vi "intialize_bottom_cam (SubVI).vi"(0 "Gain":sgl, 5 "Exposure time (ms)":sgl) -> (3 "images array out":u8[](array[numeric]), 6 "Handle out":u64, 10 "BGR out":u8[](array[numeric]), 14 "Pixel Format":u32, 15 "error out":errorcluster)   [LabVIEW 2016]
uses:
  <userlib>/Lumenera/NiLuApi.lvlibp/Controls/LuProp.ctl
  <userlib>/Lumenera/NiLuApi.lvlibp
panel:
  out "frameRate out":sgl
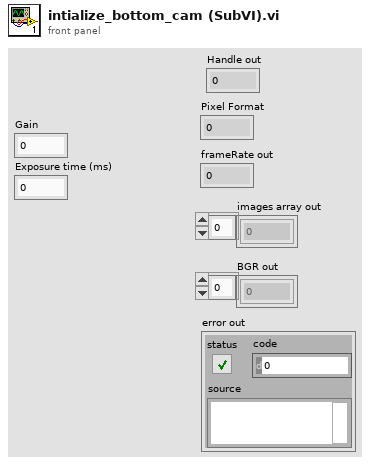
[diagram p1: front panel]
types:
  T1 = typedef "NiLuApi.lvlibp/LuProp.ctl" = u32
  T2 = cluster{"X Offset":u32, "Y Offset":u32, "Width":u32, "Heigth":u32, "Pixel Format":u32, "Bin/Sub X":u16, "FLags X":u16, "Bin/Sub Y":u16, "Flags Y":u16}
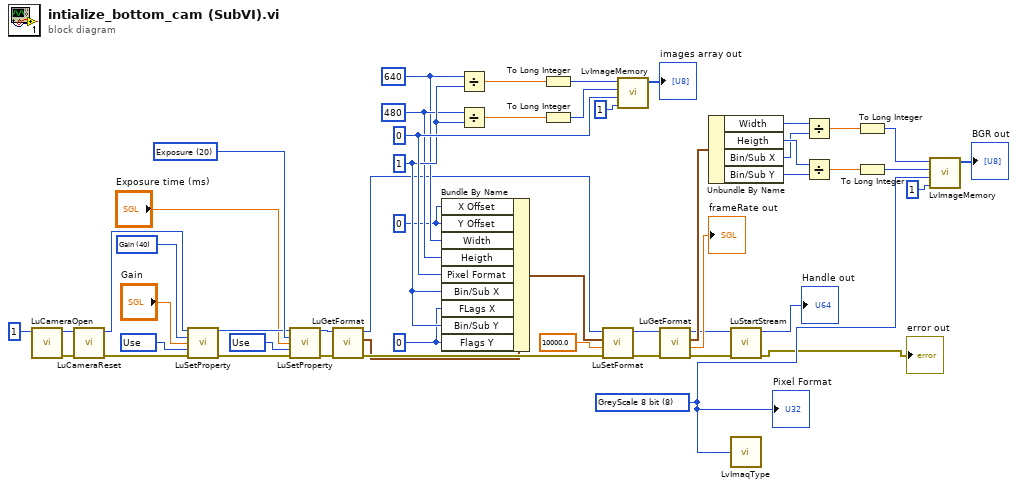
[diagram p0: block diagram]
diagram:
  w32 = u32 8 items=["8 Bit raw", "16 Bit raw", "RGB 24", "YUV422", "COUNT", "FILTER", "RGB 32", "RGB 48", "GreyScale 8 bit", "GreyScale 16 bit"] ("Pixel Format")
  w27 = u32 0 ("Pixel Format")
  w20 = u32 640 ("Width")
  w21 = u32 480 ("Heigth")
  w14 = u32 0 ("X Offset")
  w22 = u16 1 ("Bin/Sub X")
  w13 = u16 0 ("FLags X")
  w9 = -2147483648 items=["None"=0, "Use"=-2147483648, "Auto\\Master\\Little Endian"=1073741824, "Strobe From Start of Exposure"=536870912, "Polarity"=268435456, "Memory Readback"=134217728, "Unknown Maximum"=131072, "Unknown Minimum"=65536, "Red"=1, "Green1"=2, "Green2"=4, "Blue"=8] ("Capability Flag")
  w7 = T1 20 items=["Contrast"=1, "Hue"=2, "Brightness"=0, "Saturation"=3, "Sharpness"=4, "Gamma"=5, "Pan"=16, "Tilt"=17, "Roll"=18, "Zoom"=19, "Exposure"=20, "Iris"=21, "Focus"=22, "Gain"=40, "Gain Red/Magenta"=41, "Gain Blue/Cyan"=42, "Gain Green1/Yellow1"=43, "Gain Green2/Yellow2"=44, "Still Exposure"=50, "Still Gain"=51, "Red Still Gain"=52, "Green1 Still Gain"=53, "Green2 Still Gain"=54, "Blue Still Gain"=55, "Still Strobe Delay"=56, "Still Exposure Delay"=100, "Demosaicing Method"=64, "Correction Matrix"=65, "Flipping"=66, "Digital Whitebalance U"=69, "Digital Whitebalance V"=70, "Digital Gain"=71, "Digital Gain Red"=72, "Digital Gain Green"=73, "Digital Gain Blue"=74, "Color Format"=80, "Max Width"=81, "Max Height"=82, "ABS Focus"=85, "Black Level"=86, "Still Knee1 Exposure"=96, "Still Knee2 Exposure"=97, "Still Knee3 Exposure"=98, "Video Knee"=99, "Threshold"=101, "Auto Exp Target"=103, "Timestamps"=105, "Snapshot Clock Speed"=106, "Auto Exp Maximum"=107, "Temperature"=108, "Trigger"=110, "Frame Gate"=112, "Exposure Interval"=113, "PWM"=114, "Memory"=115, "Still Strobe Duration"=116, "Fan"=118, "Sync Mode"=119, "Snapshot Count"=120, "LSC X"=121, "LSC Y"=122, "Auto Iris Max"=123, "Lens Stabilization"=124, "Video Trigger"=125, "Knee2 Level"=163, "Threshold Low"=165, "Threshold High"=166, "Temperature2"=167, "Light Frequency"=168, "Luminance"=169, "Auto Gain Max"=170, "Focal Length"=174, "Iris Latency"=175, "TAP Video Configuration"=176, "TAP Still Configuration"=177, "JPEG Quality"=256, "GEV LLA"=512, "GEV DHCP"=513, "GEV PERSISTANT"=514, "GEV PERSISTANT IP Addrress"=515, "GEV PERSISTANT IP Subnet Mask"=516, "GEV PERSISTANT Default Gateway"=517, "GEV  SCPD"=518] ("Property")
  w5 = -2147483648 items=["None"=0, "Use"=-2147483648, "Auto\\Master\\Little Endian"=1073741824, "Strobe From Start of Exposure"=536870912, "Polarity"=268435456, "Memory Readback"=134217728, "Unknown Maximum"=131072, "Unknown Minimum"=65536, "Red"=1, "Green1"=2, "Green2"=4, "Blue"=8] ("Capability Flag")
  w4 = T1 40 items=["Contrast"=1, "Hue"=2, "Brightness"=0, "Saturation"=3, "Sharpness"=4, "Gamma"=5, "Pan"=16, "Tilt"=17, "Roll"=18, "Zoom"=19, "Exposure"=20, "Iris"=21, "Focus"=22, "Gain"=40, "Gain Red/Magenta"=41, "Gain Blue/Cyan"=42, "Gain Green1/Yellow1"=43, "Gain Green2/Yellow2"=44, "Still Exposure"=50, "Still Gain"=51, "Red Still Gain"=52, "Green1 Still Gain"=53, "Green2 Still Gain"=54, "Blue Still Gain"=55, "Still Strobe Delay"=56, "Still Exposure Delay"=100, "Demosaicing Method"=64, "Correction Matrix"=65, "Flipping"=66, "Digital Whitebalance U"=69, "Digital Whitebalance V"=70, "Digital Gain"=71, "Digital Gain Red"=72, "Digital Gain Green"=73, "Digital Gain Blue"=74, "Color Format"=80, "Max Width"=81, "Max Height"=82, "ABS Focus"=85, "Black Level"=86, "Still Knee1 Exposure"=96, "Still Knee2 Exposure"=97, "Still Knee3 Exposure"=98, "Video Knee"=99, "Threshold"=101, "Auto Exp Target"=103, "Timestamps"=105, "Snapshot Clock Speed"=106, "Auto Exp Maximum"=107, "Temperature"=108, "Trigger"=110, "Frame Gate"=112, "Exposure Interval"=113, "PWM"=114, "Memory"=115, "Still Strobe Duration"=116, "Fan"=118, "Sync Mode"=119, "Snapshot Count"=120, "LSC X"=121, "LSC Y"=122, "Auto Iris Max"=123, "Lens Stabilization"=124, "Video Trigger"=125, "Knee2 Level"=163, "Threshold Low"=165, "Threshold High"=166, "Temperature2"=167, "Light Frequency"=168, "Luminance"=169, "Auto Gain Max"=170, "Focal Length"=174, "Iris Latency"=175, "TAP Video Configuration"=176, "TAP Still Configuration"=177, "JPEG Quality"=256, "GEV LLA"=512, "GEV DHCP"=513, "GEV PERSISTANT"=514, "GEV PERSISTANT IP Addrress"=515, "GEV PERSISTANT IP Subnet Mask"=516, "GEV PERSISTANT Default Gateway"=517, "GEV  SCPD"=518] ("Property")
  n1 = call <userlib>:"LuCameraOpen.vi"("Camera Index"=u32 1) -> ("error out"=w47:errorcluster, "Camera handle out"=w48:u64)  [unwired: 9 in]
  n2 = call <userlib>:"LuCameraReset.vi"("error in"=w47, "Camera handle"=w48) -> ("error out"=w51:errorcluster, "Camera handle out"=w50:u64)  [unwired: 8 in]
  n3 = call <userlib>:"LuSetProperty.vi"("handle in"=w50, "Property"=w4, "value"="Gain", "Capability Flag"=w5, "error in (no error)"=w51) -> ("Handle out"=w6:u64, "error out"=w8:errorcluster)  [unwired: 9 in]
  n4 = call <userlib>:"LuSetProperty.vi"("handle in"=w6, "Property"=w7, "value"="Exposure time (ms)", "Capability Flag"=w9, "error in (no error)"=w8) -> ("Handle out"=w10:u64, "error out"=w11:errorcluster)  [unwired: 9 in]
  n5 = call <userlib>:"LuGetFormat.vi"("error in (no error)"=w11, "handle in"=w10) -> ("error out"=w18:errorcluster, "Frame Format"=w12:T2, "Handle out"=w15:u64)  [unwired: 4 in, 1 out]
  n6 = Bundle By Name(cluster=w12, "X Offset"=w14, "Y Offset"=w14, "Width"=w20, "Heigth"=w21, "Pixel Format"=w27, "Bin/Sub X"=w22, "FLags X"=w13, "Bin/Sub Y"=w22, "Flags Y"=w13) -> (w16:T2)
  n7 = Divide(x=w20, y=w22) -> (x/y=w23:dbl)
  n8 = Divide(x=w21, y=w22) -> (x/y=w24:dbl)
  n9 = To Long Integer(number=w23) -> (32bit integer=w28:i32)
  n10 = To Long Integer(number=w24) -> (32bit integer=w29:i32)
  n11 = call <userlib>:"LuSetFormat.vi"("error in (no error)"=w18, "frameRate"=sgl 10000.0, "Frame Format"=w16, "handle in"=w15) -> ("error out"=w33:errorcluster, "Handle out"=w34:u64)  [unwired: 6 in]
  n12 = call <userlib>:"LvImageMemory.vi"("Nb Images"=1, "Pixel Format"=w27, "Image height"=w29, "Image width"=w28) -> ("images array"=→"images array out":u8[])  [unwired: 7 in]
  n13 = call <userlib>:"LuGetFormat.vi"("error in (no error)"=w33, "handle in"=w34) -> ("error out"=w35:errorcluster, "frameRate out"=→"frameRate out":sgl, "Frame Format"=w37:T2, "Handle out"=w36:u64)  [unwired: 4 in]
  n14 = Unbundle By Name(w37) -> ("Width"=w38:u32, "Heigth"=w43:u32, "Bin/Sub X"=w39:u16, "Bin/Sub Y"=w44:u16)
  n15 = call <userlib>:"LuStartStream.vi"("error in"=w35, "handle in"=w36) -> ("error out"=→"error out":errorcluster, "Handle out"=→"Handle out":u64)  [unwired: 8 in]
  n16 = call <userlib>:"LvImaqType.vi"("Pixel Format"=w32) -> ()  [unwired: 1 out]
  n17 = Divide(x=w38, y=w39) -> (x/y=w40:dbl)
  n18 = Divide(x=w43, y=w44) -> (x/y=w42:dbl)
  n19 = To Long Integer(number=w40) -> (32bit integer=w41:i32)
  n20 = To Long Integer(number=w42) -> (32bit integer=w45:i32)
  n21 = call <userlib>:"LvImageMemory.vi"("Nb Images"=1, "Pixel Format"=w32, "Image height"=w45, "Image width"=w41) -> ("images array"=→"BGR out":u8[])  [unwired: 7 in]
  "Pixel Format" <- w32
